vi "Configure Sense Mode.vi"(8 "error in (no error)":errorcluster, 9 "Power Sensing Mode (0: Internal)":i32(ring) items=["Internal", "External"], 10 "Channel (1)":string="1", 11 "VISA resource name":refnum<visa-resource-name>) -> (0 "error out":errorcluster, 3 "VISA resource name out":refnum<visa-resource-name>)   [LabVIEW 2020, in "Keysight E36300 Series.lvlib"]
doc: "Configures the power supported sensing mode.\n\n<b>Note: </b>\nThis VI is only applicable for E36312A and E36313A models."
uses:
  Keysight E36300 Series.lvlib
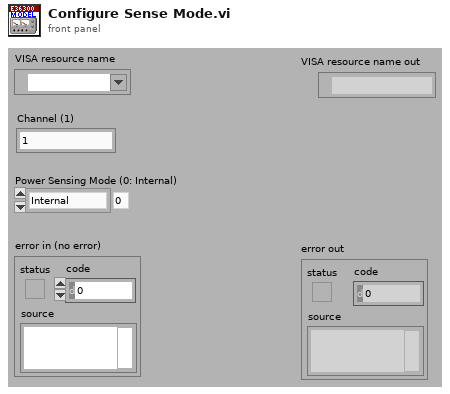
[diagram p1: front panel]
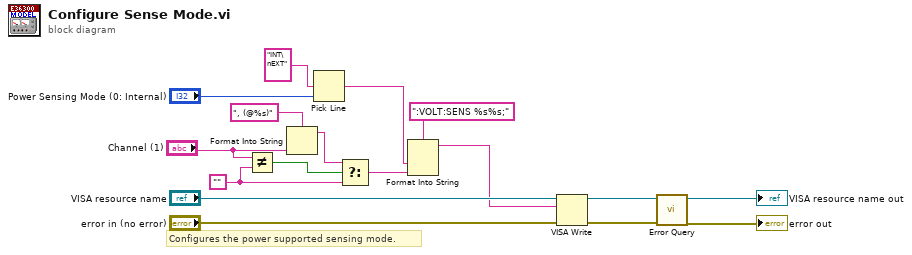
[diagram p0: block diagram]
diagram:
  w2 = ""
  # "Configures the power supported sensing mode."
  n1 = Not Equal?(x="Channel (1)", y=w2) -> (x != y?=w4:bool)
  n2 = Format Into String(format string=", (@%s)", "Channel (1)") -> (resulting string=w5:string)  [unwired: 2 in, 1 out]
  n3 = Pick Line(multi-line string="INT\nEXT", line index="Power Sensing Mode (0: Internal)") -> (output string=w14:string)  [unwired: 1 in]
  n4 = Select(t=w5, s=w4, f=w2) -> (s? t:f=w3:string)
  n5 = Format Into String(format string=":VOLT:SENS %s%s;", w14, w3) -> (resulting string=w7:string)  [unwired: 2 in, 1 out]
  n6 = VISA Write(VISA resource name="VISA resource name", write buffer=w7, error in (no error)="error in (no error)") -> (VISA resource name out=w11:refnum<visa-resource-name>, error out=w10:errorcluster)  [unwired: 1 out]
  n7 = call "Error Query.vi"("error in (no error)"=w10, "VISA resource name"=w11) -> ("error out"=→"error out":errorcluster, "VISA resource name out"=→"VISA resource name out":refnum<visa-resource-name>)  [unwired: 6 in, 2 out]
